vi "Close.vi"(8 "error in":errorcluster, 11 "Cycler Cluster.lvclass in":refnum<class "Cycler Cluster.lvclass">) -> (0 "error out":errorcluster)   [LabVIEW 2023, in "Cycler Cluster.lvclass"]
uses:
  Cycler Cluster.lvclass
  Cycler Cluster.lvclass/Cycler Cluster.ctl
  <vilib>/ADAS Replay HIL/AdasHilServices/AdasHilChannelServices.lvlib
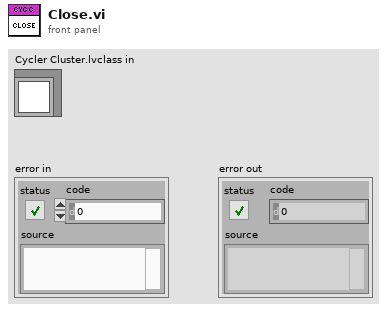
[diagram p1: front panel]
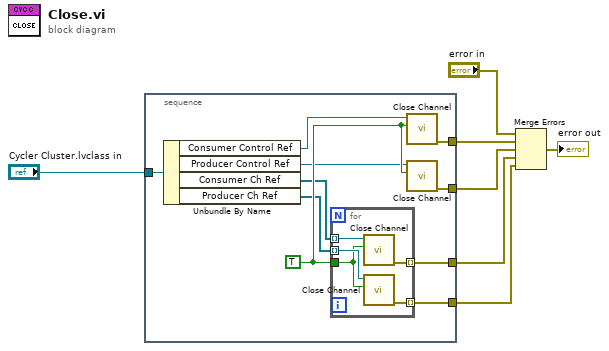
[diagram p0: block diagram]
diagram:
  n1 = stacked-sequence {
    tunnel: "Cycler Cluster.lvclass in" -> [w12]
    tunnel: [w11] -> w4
    tunnel: [w10] -> w3
    tunnel: [w9] -> w2
    tunnel: [w8] -> w1
    frame #0 {
      w17 = TRUE ("Force Destroy? (F)")
      n2 = Unbundle By Name(w12) -> ("Consumer Control Ref"=w13:refnum<k21>, "Producer Control Ref"=w14:refnum<k21>, "Consumer Ch Ref"=w15:refnum<k21>[], "Producer Ch Ref"=w16:refnum<k21>[])
      n3 = for {
        tunnel: w15 -> [w22] mode=indexing
        tunnel: w16 -> [w21] mode=indexing
        tunnel: w17 -> [w20]
        tunnel: [w19] -> w9 mode=indexing
        tunnel: [w18] -> w8 mode=indexing
        n4 = call <vilib>:"Close Channel.vi"("Force Destroy? (F)"=w20, "ADAS HIL Channel"=w22) -> ("error out"=w19:errorcluster)  [unwired: 9 in]
        n5 = call <vilib>:"Close Channel.vi"("Force Destroy? (F)"=w20, "ADAS HIL Channel"=w21) -> ("error out"=w18:errorcluster)  [unwired: 9 in]
      }
      n6 = call <vilib>:"Close Channel.vi"("Force Destroy? (F)"=w17, "ADAS HIL Channel"=w13) -> ("error out"=w11:errorcluster)  [unwired: 9 in]
      n7 = call <vilib>:"Close Channel.vi"("Force Destroy? (F)"=w17, "ADAS HIL Channel"=w14) -> ("error out"=w10:errorcluster)  [unwired: 9 in]
    }
  }
  n8 = Merge Errors("error in", w4, w3, w2, w1) -> (→"error out":errorcluster)
